vi "SUB_TP_Array_Search.vi"(2 "Search Array Name":string, 3 "Source record(s)":T1(array[cluster])) -> (1 "Desired Array":T2)   [LabVIEW 2011]
panel:
  out "record(s)":T1(array[cluster])
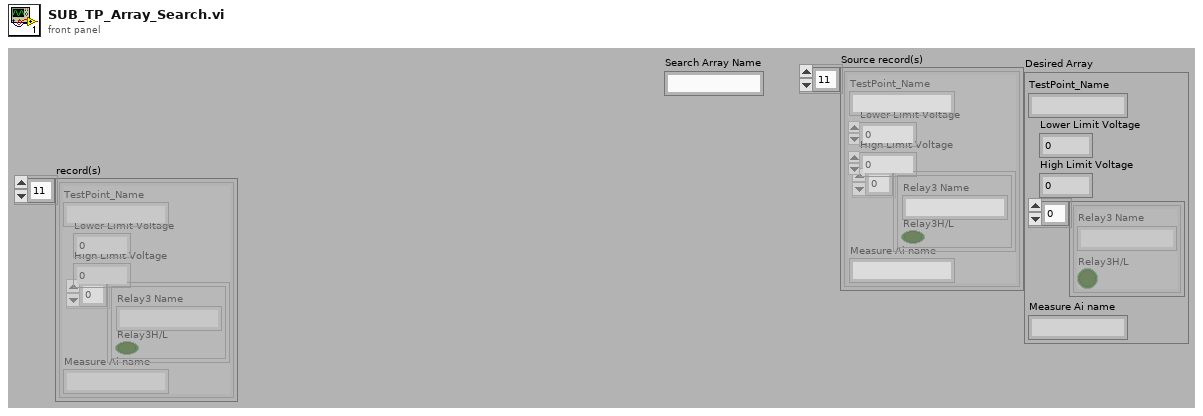
[diagram p1: front panel]
types:
  T1 = cluster{"TestPoint_Name":string, "Lower Limit Voltage":dbl, "High Limit Voltage":dbl, cluster{"Relay3 Name":string, "Relay3H/L":bool}[], "Measure Ai name":string}[]
  T2 = cluster{"TestPoint_Name":string, "Lower Limit Voltage":dbl, "High Limit Voltage":dbl, cluster{"Relay3 Name":string, "Relay3H/L":bool}[], "Measure Ai name":string}
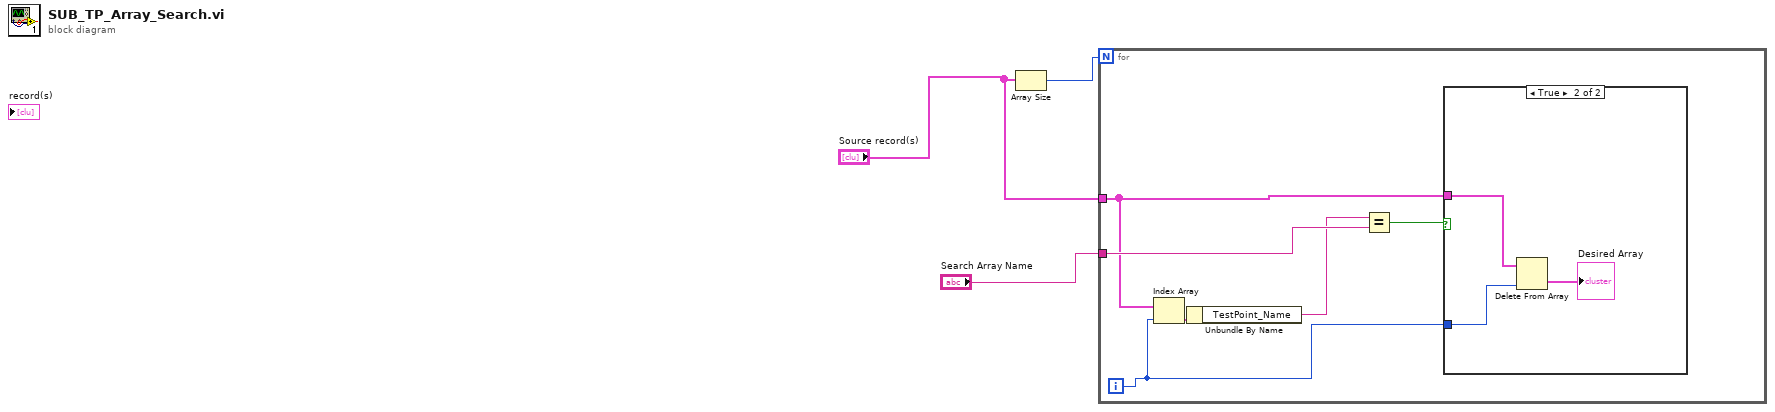
[diagram p0: block diagram]
diagram:
  n1 = Array Size(array="Source record(s)") -> (size(s)=w3:i32)
  n2 = for {
    N: w3 -> [_]
    tunnel: "Source record(s)" -> [w5]
    tunnel: "Search Array Name" -> [w8]
    i -> [w4]
    n3 = Index Array(array=w5, index=w4) -> (element=w9:T2)
    n4 = Unbundle By Name(w9) -> ("TestPoint_Name"=w7:string)
    n5 = Equal?(x=w7, y=w8) -> (x = y?=w6:bool)
    n6 = case shown="True" w6 {
      tunnel: w5 -> [_ w12]
      tunnel: w4 -> [_ w11]
      frame False {
      }
      frame True {
        n7 = Delete From Array(array=w12, index=w11) -> (deleted portion=→"Desired Array":T2)  [unwired: 1 in, 1 out]
      }
    }
  }
